vi "Read Message.vi"(8 "error in (no error)":errorcluster, 11 "Dialog in":refnum<class "Dialog.lvclass">) -> (0 "error out":errorcluster, 2 "Message":string, 3 "Dialog out":refnum<class "Dialog.lvclass">)   [LabVIEW 2012, in "Dialog.lvlib" / "Dialog.lvclass"]
doc: "Accessor VI for Dialog class."
uses:
  Dialog.lvclass
  Dialog.lvclass/Dialog.ctl
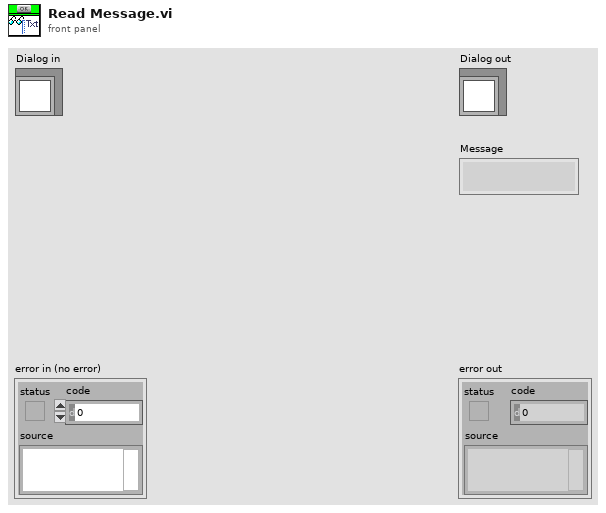
[diagram p1: front panel]
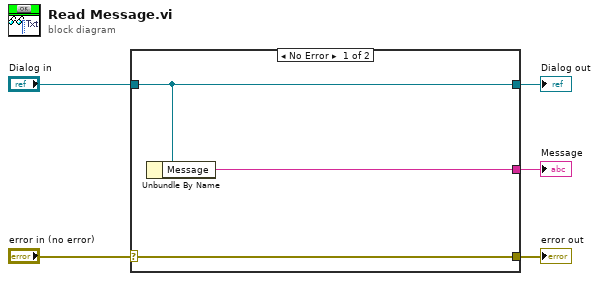
[diagram p0: block diagram]
diagram:
  n1 = case shown="No Error" "error in (no error)" {
    selector: "error in (no error)" -> [w8 w9]
    tunnel: [w8 w9] -> w4
    tunnel: [w7 w10] -> w2
    tunnel: "Dialog in" -> [w7 w10]
    tunnel: [w6 _] -> w1
    frame No Error {
      n2 = Unbundle By Name(w7) -> ("Message"=w6:string)
    }
    frame Error {
    }
  }
  "error out" <- w4
  "Dialog out" <- w2
  "Message" <- w1
